vi "IRISS V2 Joint Ref Follow.vi"(6 "error in":errorcluster, 7 "Digital Cmd [0-78]":i8, 9 "FPGA VI Reference In":refnum<k20>) -> (0 "error out":errorcluster, 3 "FPGA VI Reference Out":refnum<k20>)   [LabVIEW 2016]
uses:
  Subsystems/Global Variables.vi
  <vilib>/Utility/error.llb/Error Cluster From Error Code.vi
  <vilib>/rvi/errors/niLvFpgaAdjustHostInterfaceError.vi
  <vilib>/rvi/interface/nirviReadWriteControl/nirviReadWriteControl.xnode
  FPGA Bitfiles/PhantomControlPI_FPGATarget_QuadCtr2_E2412E44.lvbitx
  IRISS_FPGA_IO.vi
  NiFpgaLv.dll
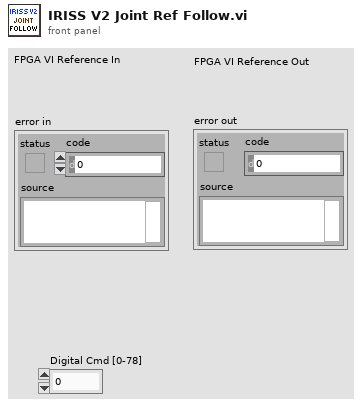
[diagram p1: front panel]
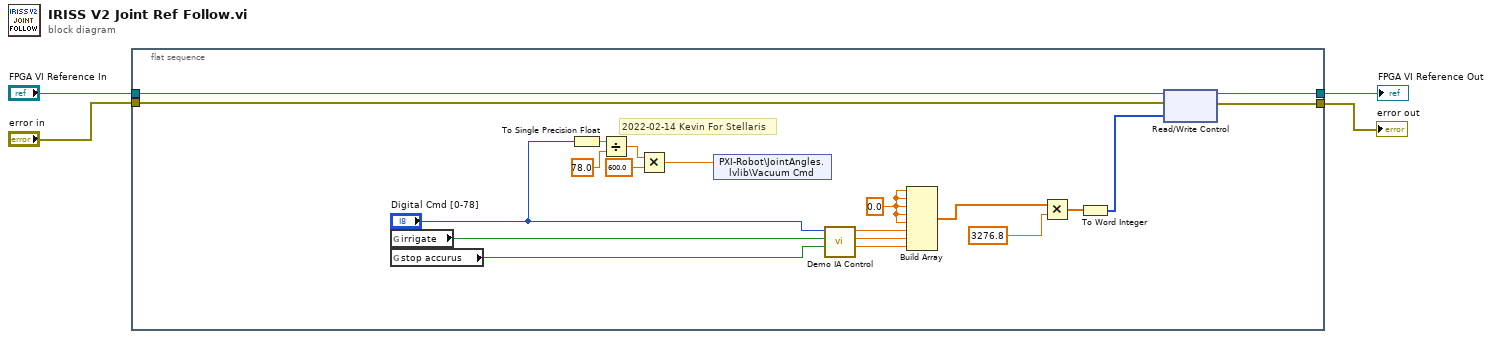
[diagram p0: block diagram]
diagram:
  n1 = flat-sequence {
    tunnel: "FPGA VI Reference In" -> [w24]
    tunnel: "error in" -> [w23]
    tunnel: [w22] -> w2
    tunnel: [w21] -> w1
    frame #0 {
      w16 = 0.0 ("element")
      # "2022-02-14 Kevin For Stellaris"
      n2 = global read "Global Variables.vi" "irrigate"() -> (w18:bool)
      n3 = global read "Global Variables.vi" "stop accurus"() -> (w17:bool)
      n4 = To Single Precision Float(number="Digital Cmd [0-78]") -> (single precision float=w10:sgl)
      n5 = Divide(x=w10, y=sgl 78.0) -> (x/y=w8:sgl)
      n6 = Multiply(x=w8, y=sgl 600.0) -> (x*y=w5:sgl)
      n7 = shared-variable "PXI-Robot\\JointAngles.lvlib\\Vacuum Cmd"(w5) -> ()  [unwired: 1 in, 1 out]
      n8 = call "Demo IA Control.vi"("E-Stop Vacuum"=w17, "Irrigate?"=w18, "8bit integer"="Digital Cmd [0-78]") -> ("Accurus Engaged Vout"=w13:dbl, "Accurus ChB Vout"=w14:dbl, "Accurus ChA Vout"=w15:dbl)  [unwired: 6 in]
      n9 = Build Array(w16, w16, w16, w16, w16, w15, w14, w13) -> (w12:dbl[])
      n10 = Multiply(x=w12, y=3276.8) -> (x*y=w20:dbl[])
      n11 = To Word Integer(number=w20) -> (16bit integer=w11:i16[])
      n12 = xnode "Read/Write Control"("FPGA VI Reference In"=w24, "error in"=w23, "AO"=w11) -> ("FPGA VI Reference Out"=w22:refnum<k20>, "error out"=w21:errorcluster)
    }
  }
  "error out" <- w1
  "FPGA VI Reference Out" <- w2
